vi "GEA2 Script Test SLB.vi"(0 "GEA2 Reference In":refnum<k24>, 1 "Version Query (for log header)":T2={"Source"=228, "Destination"=0, "Command"=1, "Message"=""} {"Command" format="%02x"; "Destination" format="%02x"; "Source" format="%02x"}, 2 "Enqueue Sends?":bool, 5 "Standalone":bool, 7 "Script path":path, 9 "Log File Path (empty for prompt)":path, 11 "Error In":errorcluster) -> (4 "GEA2 Reference Out":refnum<k24>, 6 "Pass/Fail?":bool, 8 "Report Text":string, 15 "Error Out":errorcluster)   [LabVIEW 2014]
doc: "This VI measures the time between the double line break closing and a burner relay closing."
uses:
  C:/Automation/DLLs/PC Tools .NET/GeaCommunication.dll
  Automation/DLLs/PC Tools .NET/GeaCommunication.dll
  type defs/Data In.ctl
  typedefs/Script Info.ctl
  type defs/Data Out.ctl
  library/GEA2_Toolkit.lvlib
panel:
  out "Script Info":T1 {"Overall Script File Progress" scale=0.0..1.0; "Elapsed time (s)" format="%#.1f"; "Current Script Progress" scale=0.0..1.0}
  in  "stop":bool
  in  "Board Index":i32
  in  "Default wait time (sec)":dbl=0.25 format="%#_13g"
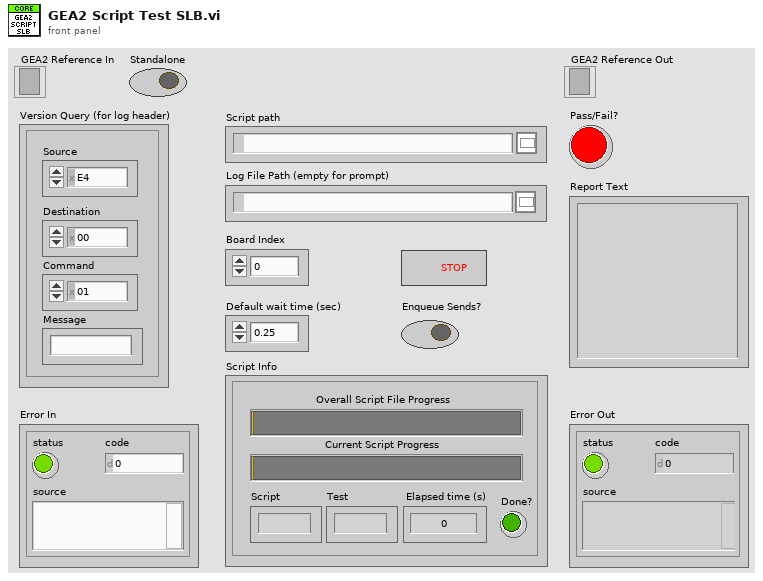
[diagram p1: front panel]
types:
  T1 = typedef "Script Info.ctl" = cluster{"Overall Script File Progress":dbl, "Current Script Progress":dbl, "Script":string, "Test":string, "Elapsed time (s)":dbl, "Done?":bool}
  T2 = typedef "GEA2_Toolkit.lvlib/Data In.ctl" = cluster{"Source":u8, "Destination":u8, "Command":u8, "Message":string}
  T3 = enum16{"open", "replace", "create", "open or create", "replace or create", "replace or create with confirmation"}
  T4 = typedef "GEA2_Toolkit.lvlib/Data Out.ctl" = cluster{"Source":u8, "Destination":u8, "Command":u8, "Length":u8, "CRC":u16, "Message":string}
  T5 = typedef "Script Output.ctl" = cluster{"Command Data":string[], "Command Type":T6[], "Test Name":string, "Wait Time (s)":dbl[], "Continue if failed?":bool[]}
  T6 = typedef "Command Type.ctl" = enum16{"WRITE", "READ", "ERDWRITE", "ERDREAD"}
  T7 = typedef "GEA2_Toolkit.lvlib/Source_Destination.ctl" = cluster{"Source":u8, "Destination":u8}
  T8 = typedef "GEA2_Toolkit.lvlib/ERD Write Data In.ctl" = cluster{"ERD Number":u16, "Data Type":enum16{"string", "boolean", "uint8_t", "uint16_t", "uint32_t"}, "Data":string}
  T9 = typedef "GEA2_Toolkit.lvlib/ERD Read Data In.ctl" = cluster{"ERD Number":u16, "Data Type":enum16{"string", "boolean", "uint8_t", "uint16_t", "uint32_t", "uint64_t"}}
  T10 = typedef "GEA2_Toolkit.lvlib/ERD Read Data Out.ctl" = cluster{"ERD Number":u16, "Data":string}
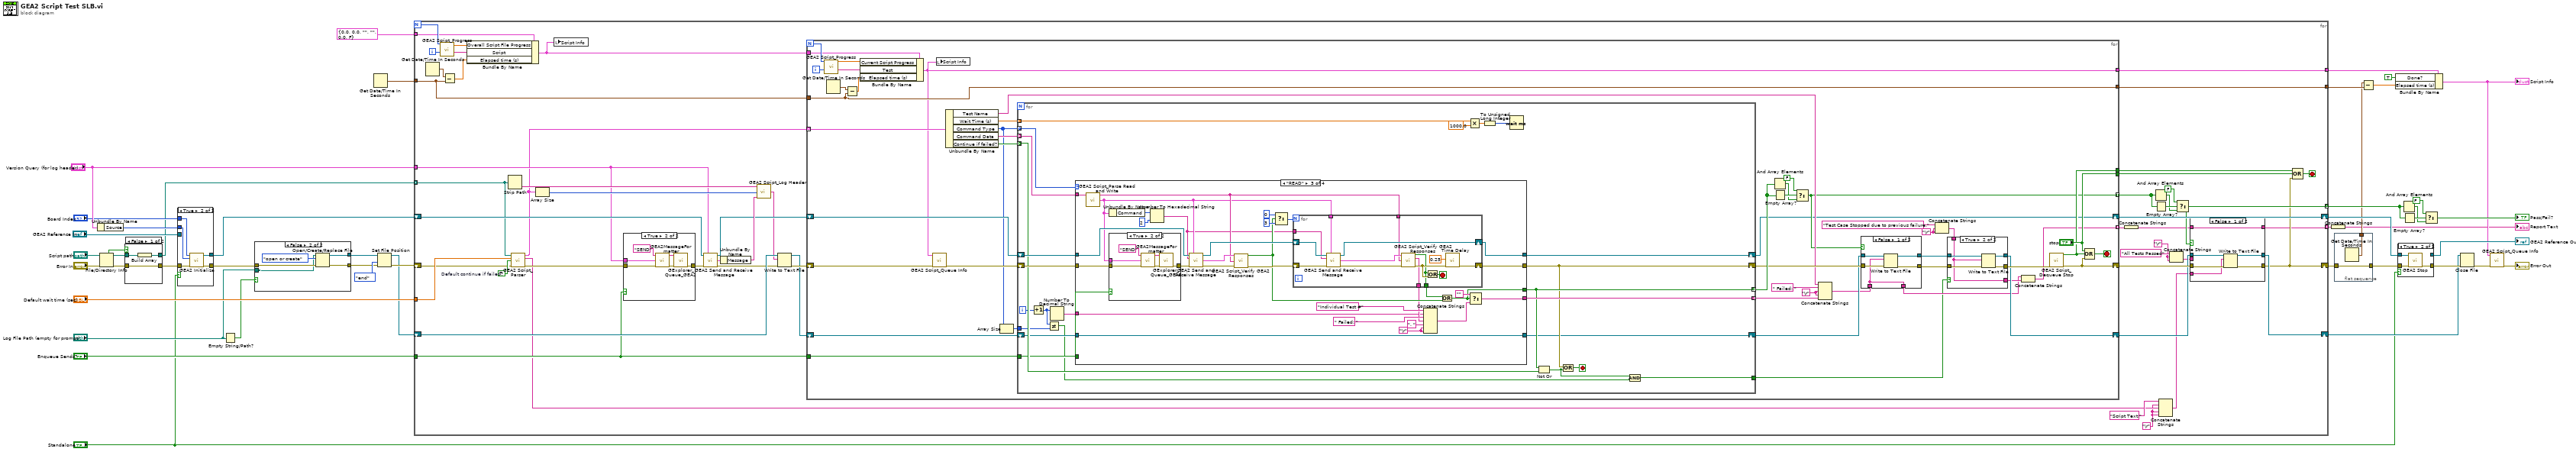
[diagram p0: block diagram]
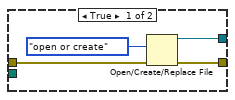
[diagram p2: hidden frame]
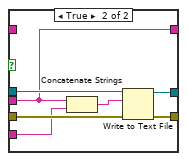
[diagram p4: hidden frame]
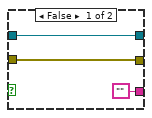
[diagram p5: hidden frame]
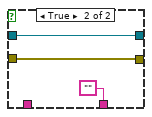
[diagram p6: hidden frame]
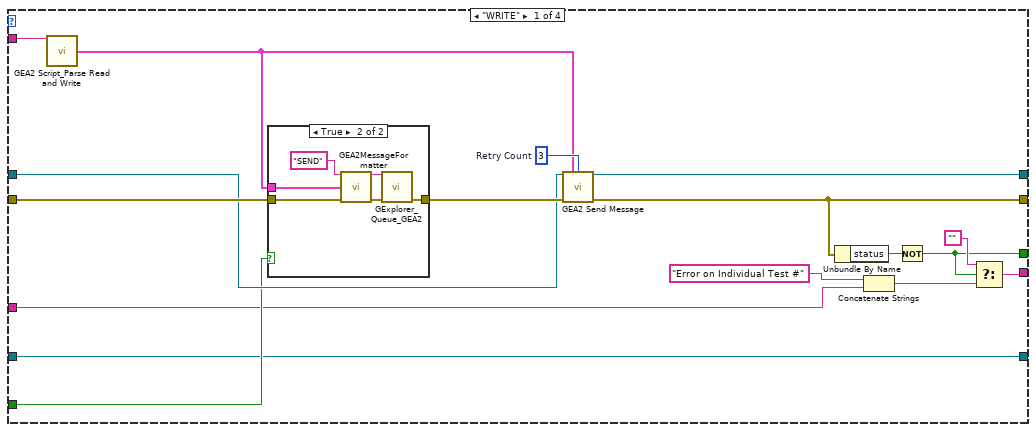
[diagram p7: hidden frame]
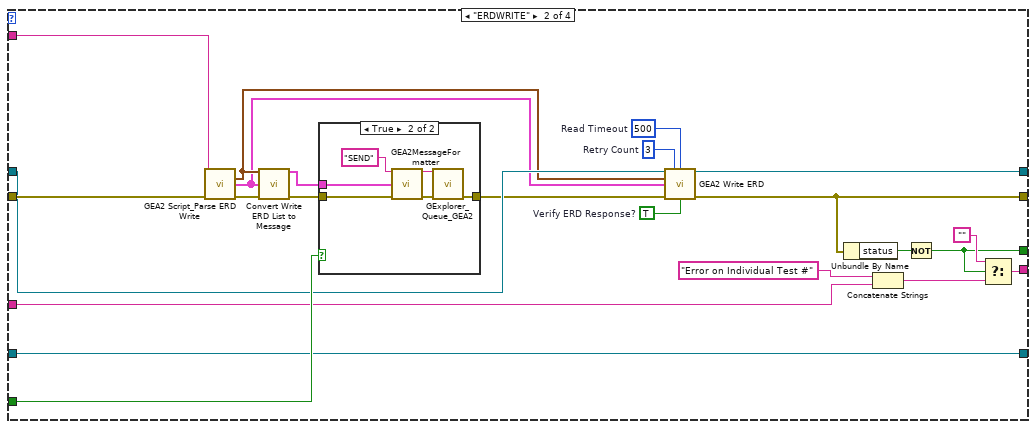
[diagram p9: hidden frame]
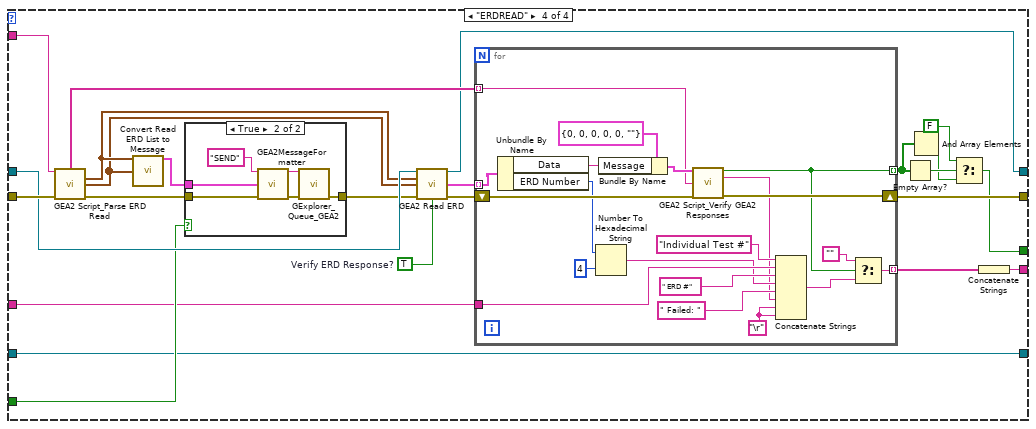
[diagram p12: hidden frame]
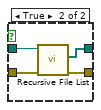
[diagram p15: hidden frame]
diagram:
  n1 = Unbundle By Name("Version Query (for log header)") -> ("Source"=w37:u8)
  n2 = File/Directory Info(path="Script path", error in="Error In") -> (path out=w41:path, directory=w40:bool, error out=w42:errorcluster)  [unwired: 4 out]
  n3 = case shown="False" w40 {
    tunnel: w42 -> [w47 w53]
    tunnel: w41 -> [w49 w52]
    tunnel: [w48 w51] -> w35
    tunnel: [w47 w50] -> w39
    frame False {
      n4 = Build Array(w49) -> (w48:path[])
    }
    frame True {
      n5 = call <vilib>:"Recursive File List.vi"("error in (no error)"=w53, "Folder Path"=w52) -> ("error out"=w50:errorcluster, "All Files in Dir"=w51:path[])  [unwired: 5 in, 3 out]
    }
  }
  n6 = case shown="True" "Standalone" {
    tunnel: [w55 w60] -> w29
    tunnel: [w54 w59] -> w32
    tunnel: "Board Index" -> [_ w57]
    tunnel: w37 -> [_ w58]
    tunnel: w39 -> [w55 w56]
    tunnel: "GEA2 Reference In" -> [w54 _]
    frame False {
    }
    frame True {
      n7 = call "GEA2 Initialize.vi"("Board Index"=w57, "Source Address"=w58, "error in"=w56) -> ("GEA2 Reference Out"=w59:refnum<k24>, "error out"=w60:errorcluster)  [unwired: 10 in, 1 out]
    }
  }
  n8 = Empty String/Path?(string/path="Log File Path (empty for prompt)") -> (empty?=w30:bool)
  n9 = case shown="False" w30 {
    tunnel: w29 -> [w63 w68]
    tunnel: [w62 w67] -> w27
    tunnel: [w61 w66] -> w26
    tunnel: "Log File Path (empty for prompt)" -> [_ w65]
    frame True {
      n10 = Open/Create/Replace File(error in=w63, operation (0:open)=T3."open or create") -> (refnum out=w62:refnum<file>, error out=w61:errorcluster)  [unwired: 4 in, 1 out]
    }
    frame False {
      n11 = Open/Create/Replace File(file path (use dialog)=w65, error in=w68, operation (0:open)=T3."open or create") -> (refnum out=w67:refnum<file>, error out=w66:errorcluster)  [unwired: 3 in, 1 out]
    }
  }
  n12 = Get Date/Time In Seconds() -> (seconds since 1Jan1904=w14:timestamp)
  n13 = Set File Position(refnum=w27, from (0:start)=enum16{"start", "end", "current"}."end", error in=w26) -> (refnum out=w24:refnum<file>, error out=w25:errorcluster)  [unwired: 1 in]
  n14 = for {
    N -> [w86]
    tunnel: "Default wait time (sec)" -> [w123]
    tunnel: "Version Query (for log header)" -> [w92]
    shift-right: [w91] -> w13
    shift-left: w25 -> [w116]
    shift-right: [w106] -> w33
    shift-left: w32 -> [w114]
    tunnel: w35 -> [w113] mode=indexing
    tunnel: "Enqueue Sends?" -> [w107]
    shift-right: [w103] -> w21
    shift-left: w24 -> [w112]
    tunnel: [w93] -> w17 mode=indexing
    tunnel: T1 {"Overall Script File Progress"=0.0, "Current Script Progress"=0.0, "Script"="", "Test"="", "Elapsed time (s)"=0.0, "Done?"=FALSE} ("Script Info") -> [w85]
    tunnel: w14 -> [w80]
    tunnel: [w79] -> w11
    tunnel: [w78] -> w9
    tunnel: [w73] -> w3 mode=indexing
    i -> [w87]
    stop <- w90 stop-if-true
    w74 = "\r"
    w70 = "\r"
    w117 = TRUE  # Default continue if failed?
    n15 = Get Date/Time In Seconds() -> (seconds since 1Jan1904=w84:timestamp)
    n16 = call "GEA2 Script_Progress.vi"("Total iterations"=w86, "Current iteration"=w87) -> ("Completion percent"=w82:dbl, "Current test"=w81:string)  [unwired: 12 in]
    n17 = Subtract(x=w84, y=w80) -> (x-y=w83:dbl)
    n18 = Bundle By Name(cluster=w85, "Overall Script File Progress"=w82, "Script"=w81, "Elapsed time (s)"=w83) -> (w77:T1)
    n19 = Strip Path(path=w113) -> (name=w122:string)  [unwired: 1 out]
    n20 = call "GEA2 Script_Parser.vi"("Script path"=w113, "Default wait time (sec)"=w123, "Default continue if failed?"=w117, "Error In"=w116) -> ("Script Output"=w71:T5[], "GEA2 Script"=w101:string, "Error Out"=w115:errorcluster)  [unwired: 9 in]
    n21 = Array Size(array=w71) -> (size(s)=w121:i32)
    n22 = local write "Script Info"(w77) -> ()
    n23 = case shown="True" w107 {
      tunnel: w92 -> [_ w386]
      tunnel: [w383 w385] -> w120
      tunnel: w115 -> [w383 w384]
      frame False {
      }
      frame True {
        n24 = call "GEA2MessageFormatter.vi"("Prefix(Send/Recv)"="SEND", "GEA2 Data In"=w386, "Error In"=w384) -> ("Output String"=w389:string, "Error Out"=w388:errorcluster)  [unwired: 11 in]
        n25 = call "GExplorer_Queue_GEA2.vi"("Output String"=w389, "error in (no error)"=w388) -> ("error out"=w385:errorcluster)  [unwired: 13 in]
      }
    }
    n26 = call "GEA2 Send and Receive Message.vi"("GEA2 Reference In"=w114, "Input Data"=w92, "Error In"=w120) -> ("GEA2 Reference Out"=w109:refnum<k24>, "Converted Data Out"=w119:T4, "Error Out"=w111:errorcluster)  [unwired: 9 in, 1 out]
    n27 = Unbundle By Name(w119) -> ("Message"=w118:string)
    n28 = call "GEA2 Script_Log Header.vi"("Filename"=w122, "# of Test Cases"=w121, "Version"=w118) -> ("Header"=w76:string)  [unwired: 12 in]
    n29 = Write to Text File(file (use dialog)=w112, text=w76, error in=w111) -> (refnum out=w108:refnum<file>, error out=w110:errorcluster)  [unwired: 1 in, 1 out]
    n30 = for {
      N -> [w170]
      tunnel: [w142] -> w75 mode=indexing
      tunnel: [w147] -> w96 mode=indexing
      shift-right: [w137] -> w105
      shift-left: w110 -> [w164]
      tunnel: w71 -> [w176] mode=indexing
      shift-right: [w146] -> w106
      shift-left: w109 -> [w162]
      shift-right: [w148] -> w104
      shift-left: w108 -> [w174]
      tunnel: w107 -> [w175]
      tunnel: ["stop"] -> w88
      tunnel: [w171] -> w89
      tunnel: w77 -> [w169]
      tunnel: w80 -> [w161]
      tunnel: [w161] -> w79
      tunnel: [w160] -> w78
      i -> [w141]
      stop <- w173 stop-if-true
      w151 = "\r"
      w155 = "\r"
      n31 = call "GEA2 Script_Progress.vi"("Total iterations"=w170, "Current iteration"=w141) -> ("Completion percent"=w167:dbl, "Current test"=w168:string)  [unwired: 12 in]
      n32 = Get Date/Time In Seconds() -> (seconds since 1Jan1904=w166:timestamp)
      n33 = Subtract(x=w166, y=w161) -> (x-y=w165:dbl)
      n34 = Bundle By Name(cluster=w169, "Current Script Progress"=w167, "Test"=w168, "Elapsed time (s)"=w165) -> (w160:T1)
      n35 = call "GEA2 Script_Queue Info.vi"("Script Info"=w160, "error in (no error)"=w164) -> ("error out"=w163:errorcluster)  [unwired: 13 in]
      n36 = local write "Script Info"(w160) -> ()
      n37 = Unbundle By Name(w176) -> ("Test Name"=w157:string, "Wait Time (s)"=w183:dbl[], "Command Type"=w140:T6[], "Command Data"=w184:string[], "Continue if failed?"=w182:bool[])
      n38 = Array Size(array=w140) -> (size(s)=w139:i32)
      n39 = for {
        shift-right: [w209] -> w159
        shift-left: w163 -> [w223]
        shift-right: [w214] -> w146
        shift-left: w162 -> [w222]
        tunnel: w140 -> [w224] mode=indexing
        tunnel: w184 -> [w221] mode=indexing
        tunnel: w183 -> [w218] mode=indexing
        tunnel: w182 -> [w220] mode=indexing
        tunnel: [w213] -> w181 mode=indexing
        tunnel: [w212] -> w177 mode=indexing
        tunnel: w175 -> [w219]
        shift-right: [w208] -> w158
        shift-left: w174 -> [w211]
        tunnel: w139 -> [w204]
        tunnel: [w201] -> w138
        i -> [w207]
        stop <- w210 stop-if-true
        n40 = Increment(x=w207) -> (x+1=w205:i32)
        n41 = Not Equal?(x=w205, y=w204) -> (x != y?=w203:bool)
        n42 = Number To Decimal String(number=w205) -> (decimal integer string=w206:string)  [unwired: 1 in]
        n43 = case shown="\"READ\"" w224 {
          tunnel: w223 -> [w238 w266 w289 w354]
          tunnel: w222 -> [w235 w263 w288 w353]
          tunnel: w221 -> [w241 w267 w310 w352]
          tunnel: [w231 w252 w301 w350] -> w209
          tunnel: [w240 w271 w302 w347] -> w214
          tunnel: [w226 w254 w293 w345] -> w213
          tunnel: [w228 w253 w291 w340] -> w212
          tunnel: w219 -> [w234 w264 w287 w336]
          tunnel: w211 -> [w233 w259 w286 w333]
          tunnel: [w233 w259 w286 w333] -> w208
          tunnel: w206 -> [w225 w249 w283 w332]
          frame "WRITE" {
            w239 = u32 3  # Retry Count
            n44 = call "GEA2 Script_Parse Read and Write.vi"("Data"=w241) -> ("GEA2 Message"=w237:T2)  [unwired: 13 in, 1 out]
            n45 = case shown="True" w234 {
              tunnel: w237 -> [_ w245]
              tunnel: [w242 w244] -> w236
              tunnel: w238 -> [w242 w243]
              frame False {
              }
              frame True {
                n46 = call "GEA2MessageFormatter.vi"("Prefix(Send/Recv)"="SEND", "GEA2 Data In"=w245, "Error In"=w243) -> ("Output String"=w248:string, "Error Out"=w247:errorcluster)  [unwired: 11 in]
                n47 = call "GExplorer_Queue_GEA2.vi"("Output String"=w248, "error in (no error)"=w247) -> ("error out"=w244:errorcluster)  [unwired: 13 in]
              }
            }
            n48 = call "GEA2 Send Message.vi"("GEA2 Reference In"=w235, "Input Data"=w237, "Retry Count"=w239, "Error In"=w236) -> ("GEA2 Reference Out"=w240:refnum<k24>, "Error Out"=w231:errorcluster)  [unwired: 10 in]
            n49 = Unbundle By Name(w231) -> ("status"=w232:bool)
            n50 = Concatenate Strings("Error on Individual Test #" ("string"), w225) -> (w227:string)
            n51 = Not(x=w232) -> (.not. x?=w228:bool)
            n52 = Select(t="", s=w228, f=w227) -> (s? t:f=w226:string)
          }
          frame "ERDWRITE" {
            w268 = TRUE  # Verify ERD Response?
            w269 = u32 500  # Read Timeout
            w270 = 3  # Retry Count
            n53 = call "GEA2 Script_Parse ERD Write.vi"("Data"=w267, "Error In"=w266) -> ("GEA Inputs"=w261:T7, "Write ERD List"=w260:T8[], "Error Out"=w251:errorcluster)  [unwired: 11 in]
            n54 = call "Convert Write ERD List to Message.vi"("GEA Inputs"=w261, "Write ERD List"=w260, "Error In"=w251) -> ("GEA Message"=w265:T2, "Error Out"=w250:errorcluster)  [unwired: 11 in]
            n55 = case shown="True" w264 {
              tunnel: w265 -> [_ w275]
              tunnel: [w272 w274] -> w262
              tunnel: w250 -> [w272 w273]
              frame False {
              }
              frame True {
                n56 = call "GEA2MessageFormatter.vi"("Prefix(Send/Recv)"="SEND", "GEA2 Data In"=w275, "Error In"=w273) -> ("Output String"=w278:string, "Error Out"=w277:errorcluster)  [unwired: 11 in]
                n57 = call "GExplorer_Queue_GEA2.vi"("Output String"=w278, "error in (no error)"=w277) -> ("error out"=w274:errorcluster)  [unwired: 13 in]
              }
            }
            n58 = call "GEA2 Write ERD.vi"("GEA2 Reference In"=w263, "Retry Count"=w270, "Read Timeout (ms)"=w269, "GEA Inputs"=w261, "Write ERD List"=w260, "Error In"=w262, "Verify ERD Response?"=w268) -> ("GEA2 Reference Out"=w271:refnum<k24>, "Error Out"=w252:errorcluster)  [unwired: 6 in, 1 out]
            n59 = Unbundle By Name(w252) -> ("status"=w258:bool)
            n60 = Concatenate Strings("Error on Individual Test #" ("string"), w249) -> (w255:string)
            n61 = Not(x=w258) -> (.not. x?=w253:bool)
            n62 = Select(t="", s=w253, f=w255) -> (s? t:f=w254:string)
          }
          frame "READ" {
            w284 = "\r"
            n63 = call "GEA2 Script_Parse Read and Write.vi"("Data"=w310) -> ("Expected Response"=w292:string, "GEA2 Message"=w282:T2)  [unwired: 13 in]
            n64 = case shown="True" w287 {
              tunnel: w282 -> [_ w314]
              tunnel: [w311 w313] -> w290
              tunnel: w289 -> [w311 w312]
              frame False {
              }
              frame True {
                n65 = call "GEA2MessageFormatter.vi"("Prefix(Send/Recv)"="SEND", "GEA2 Data In"=w314, "Error In"=w312) -> ("Output String"=w317:string, "Error Out"=w316:errorcluster)  [unwired: 11 in]
                n66 = call "GExplorer_Queue_GEA2.vi"("Output String"=w317, "error in (no error)"=w316) -> ("error out"=w313:errorcluster)  [unwired: 13 in]
              }
            }
            n67 = Unbundle By Name(w282) -> ("Command"=w281:u8)
            n68 = Number To Hexadecimal String(1:i16 2 ("width (-)"), 2:w281) -> (0:w279:string)
            n69 = call "GEA2 Send and Receive Message.vi"("GEA2 Reference In"=w288, "Input Data"=w282, "Expected Command"=w279, "Error In"=w290) -> ("GEA2 Reference Out"=w306:refnum<k24>, "Converted Data Out"=w309:T4, "Error Out"=w308:errorcluster)  [unwired: 8 in, 1 out]
            n70 = call "GEA2 Script_Verify GEA2 Responses.vi"("Actual Response"=w309, "Expected Response"=w292, "Error In"=w308) -> ("Pass/Fail?"=w299:bool, "Error Out"=w307:errorcluster)  [unwired: 10 in, 1 out]
            n71 = Select(t=0, s=w299, f=3) -> (s? t:f=w303:i32)
            n72 = for {
              N: w303 -> [_]
              shift-right: [w327] -> w301
              shift-left: w307 -> [w330]
              shift-right: [w328] -> w302
              shift-left: w306 -> [w329]
              tunnel: w292 -> [w323]
              tunnel: [w321] -> w295
              tunnel: w282 -> [w320]
              tunnel: [w319] -> w300
              tunnel: w279 -> [w318]
              stop <- w331 stop-if-true
              n73 = call "GEA2 Send and Receive Message.vi"("GEA2 Reference In"=w329, "Input Data"=w320, "Expected Command"=w318, "Error In"=w330) -> ("GEA2 Reference Out"=w328:refnum<k24>, "Converted Data Out"=w324:T4, "Error Out"=w325:errorcluster)  [unwired: 8 in, 1 out]
              n74 = call "GEA2 Script_Verify GEA2 Responses.vi"("Actual Response"=w324, "Expected Response"=w323, "Error In"=w325) -> ("Pass/Fail?"=w319:bool, "Report Text"=w321:string, "Error Out"=w322:errorcluster)  [unwired: 10 in]
              n75 = Or(x=w319, y=w322) -> (x .or. y?=w331:bool)
              n76 = call "Time Delay"("error in (no error)"=w322, "Delay Time (s)"=0.25) -> ("error out"=w327:errorcluster)  [unwired: 9 in]
            }
            n77 = Concatenate Strings("Individual Test #", w283, " Failed: " ("string"), w295, ". " ("string"), w284, w284) -> (w294:string)
            n78 = Or(x=w300, y=w299) -> (x .or. y?=w291:bool)
            n79 = Select(t="", s=w291, f=w294) -> (s? t:f=w293:string)
          }
          frame "ERDREAD" {
            w355 = TRUE  # Verify ERD Response?
            n80 = call "GEA2 Script_Parse ERD Read.vi"("Data"=w352, "Error In"=w354) -> ("Expected Responses"=w348:string[], "GEA Inputs"=w335:T7, "Read ERD List"=w334:T9[], "Error Out"=w339:errorcluster)  [unwired: 10 in]
            n81 = call "Convert Read ERD List to Message.vi"("GEA Inputs"=w335, "Read ERD List"=w334) -> ("GEA Message"=w338:T2)  [unwired: 12 in, 1 out]
            n82 = case shown="True" w336 {
              tunnel: w338 -> [_ w359]
              tunnel: [w356 w358] -> w337
              tunnel: w339 -> [w356 w357]
              frame False {
              }
              frame True {
                n83 = call "GEA2MessageFormatter.vi"("Prefix(Send/Recv)"="SEND", "GEA2 Data In"=w359, "Error In"=w357) -> ("Output String"=w362:string, "Error Out"=w361:errorcluster)  [unwired: 11 in]
                n84 = call "GExplorer_Queue_GEA2.vi"("Output String"=w362, "error in (no error)"=w361) -> ("error out"=w358:errorcluster)  [unwired: 13 in]
              }
            }
            n85 = call "GEA2 Read ERD.vi"("GEA2 Reference In"=w353, "GEA Inputs"=w335, "Read ERD List"=w334, "Error In"=w337, "Verify ERD Response?"=w355) -> ("GEA2 Reference Out"=w347:refnum<k24>, "ERD Data Out"=w349:T10[], "Error Out"=w351:errorcluster)  [unwired: 7 in, 1 out]
            n86 = for {
              shift-right: [w376] -> w350
              shift-left: w351 -> [w379]
              tunnel: w349 -> [w382] mode=indexing
              tunnel: w348 -> [w377] mode=indexing
              tunnel: [w366] -> w344 mode=indexing
              tunnel: w332 -> [w370]
              tunnel: [w365] -> w346 mode=indexing
              w363 = "\r"
              n87 = Unbundle By Name(w382) -> ("Data"=w378:string, "ERD Number"=w373:u16)
              n88 = Number To Hexadecimal String(1:i16 4 ("width (-)"), 2:w373) -> (0:w368:string)
              n89 = Bundle By Name(cluster=T4 {"Source"=0, "Destination"=0, "Command"=0, "Length"=0, "CRC"=0, "Message"=""} ("Actual Response"), "Message"=w378) -> (w380:T4)
              n90 = call "GEA2 Script_Verify GEA2 Responses.vi"("Actual Response"=w380, "Expected Response"=w377, "Error In"=w379) -> ("Pass/Fail?"=w366:bool, "Report Text"=w364:string, "Error Out"=w376:errorcluster)  [unwired: 10 in]
              n91 = Concatenate Strings("Individual Test #", w370, " ERD #", w368, " Failed: " ("string"), w364, w363, w363) -> (w375:string)
              n92 = Select(t="", s=w366, f=w375) -> (s? t:f=w365:string)
            }
            n93 = Empty Array?(array=w344) -> (empty?=w343:bool)
            n94 = And Array Elements(Boolean array=w344) -> (logical AND=w342:bool)
            n95 = Select(t=FALSE, s=w343, f=w342) -> (s? t:f=w340:bool)
            n96 = Concatenate Strings(w346) -> (w345:string)
          }
        }
        n97 = Multiply(x=w218, y=1000.0) -> (x*y=w216:dbl)
        n98 = To Unsigned Long Integer(number=w216) -> (unsigned 32bit integer=w215:u32)
        n99 = Wait (ms)(milliseconds to wait=w215) -> ()  [unwired: 1 out]
        n100 = Not Or(1:w220, 2:w212) -> (0:w202:bool)
        n101 = Or(x=w209, y=w202) -> (x .or. y?=w210:bool)
        n102 = Compound Arithmetic op=AND(w202, w203) -> (w201:bool)
      }
      n103 = And Array Elements(Boolean array=w177) -> (logical AND=w179:bool)
      n104 = Empty Array?(array=w177) -> (empty?=w180:bool)
      n105 = Select(t=FALSE, s=w180, f=w179) -> (s? t:f=w147:bool)
      n106 = Concatenate Strings(w157, " Failed: " ("string"), w155, w155, w181) -> (w145:string)
      n107 = case shown="False" w147 {
        tunnel: w159 -> [w197 w200]
        tunnel: w158 -> [w196 w199]
        tunnel: [w195 w199] -> w153
        tunnel: [w194 w200] -> w154
        tunnel: w145 -> [w193 _]
        tunnel: [w193 ""] -> w143
        frame False {
          n108 = Write to Text File(file (use dialog)=w196, text=w193, error in=w197) -> (refnum out=w195:refnum<file>, error out=w194:errorcluster)  [unwired: 1 in, 1 out]
        }
        frame True {
        }
      }
      n109 = Concatenate Strings("Test Case Stopped due to previous failure." ("string"), w151, w151) -> (w150:string)
      n110 = case shown="True" w138 {
        tunnel: w154 -> [w187 w192]
        tunnel: w153 -> [w186 w189]
        tunnel: [w186 w191] -> w148
        tunnel: [w187 w190] -> w149
        tunnel: w150 -> [_ w188]
        tunnel: ["" w188] -> w144
        frame False {
        }
        frame True {
          n111 = Write to Text File(file (use dialog)=w189, text=w188, error in=w192) -> (refnum out=w191:refnum<file>, error out=w190:errorcluster)  [unwired: 1 in, 1 out]
        }
      }
      n112 = Concatenate Strings(w143, w144) -> (w142:string)
      n113 = call "GEA2 Script_Dequeue Stop.vi"("error in (no error)"=w149) -> ("Stop Queue?"=w171:bool, "error out"=w137:errorcluster)  [unwired: 13 in]
      n114 = Compound Arithmetic op=OR("stop", w171, w137) -> (w173:bool)
    }
    n115 = Concatenate Strings(w75) -> (w72:string)
    n116 = And Array Elements(Boolean array=w96) -> (logical AND=w98:bool)
    n117 = Empty Array?(array=w96) -> (empty?=w99:bool)
    n118 = Concatenate Strings("Script Text:" ("string"), w70, w101, w70, w70) -> (w100:string)
    n119 = Concatenate Strings("All Tests Passed" ("text"), w74, w74) -> (w94:string)
    n120 = Select(t=FALSE, s=w99, f=w98) -> (s? t:f=w93:bool)
    n121 = case shown="False" w93 {
      tunnel: w105 -> [w129 w136]
      tunnel: [w126 w135] -> w91
      tunnel: w104 -> [w128 w134]
      tunnel: [w127 w133] -> w103
      tunnel: w94 -> [_ w130]
      tunnel: w100 -> [w125 w131]
      tunnel: [w124 w130] -> w73
      tunnel: w72 -> [w124 _]
      frame False {
        n122 = Write to Text File(file (use dialog)=w128, text=w125, error in=w129) -> (refnum out=w127:refnum<file>, error out=w126:errorcluster)  [unwired: 1 in, 1 out]
      }
      frame True {
        n123 = Concatenate Strings(w130, w131) -> (w132:string)
        n124 = Write to Text File(file (use dialog)=w134, text=w132, error in=w136) -> (refnum out=w133:refnum<file>, error out=w135:errorcluster)  [unwired: 1 in, 1 out]
      }
    }
    n125 = Compound Arithmetic op=OR(w89, w88, w91) -> (w90:bool)
  }
  n126 = Concatenate Strings(w3) -> (→"Report Text":string)
  n127 = flat-sequence {
    tunnel: [w391] -> w12
    tunnel: w13 -> [w391]
    tunnel: [w390] -> w10
    frame #0 {
      n128 = Get Date/Time In Seconds() -> (seconds since 1Jan1904=w390:timestamp)
    }
  }
  n129 = Subtract(x=w10, y=w11) -> (x-y=w8:dbl)
  n130 = Bundle By Name(cluster=w9, "Done?"=TRUE, "Elapsed time (s)"=w8) -> (w5:T1)
  "Script Info" <- w5
  n131 = case shown="True" "Standalone" {
    tunnel: [w393 w395] -> w22
    tunnel: w12 -> [w393 w396]
    tunnel: w33 -> [w392 w394]
    tunnel: [w392 _] -> w23
    frame False {
    }
    frame True {
      n132 = call "GEA2 Stop.vi"("GEA2 Reference In"=w394, "Error In"=w396) -> ("Error Out"=w395:errorcluster)  [unwired: 13 in]
    }
  }
  "GEA2 Reference Out" <- w23
  n133 = And Array Elements(Boolean array=w17) -> (logical AND=w19:bool)
  n134 = Empty Array?(array=w17) -> (empty?=w20:bool)
  n135 = Select(t=FALSE, s=w20, f=w19) -> (s? t:f=→"Pass/Fail?":bool)
  n136 = Close File(refnum=w21, error in=w22) -> (error out=w6:errorcluster)  [unwired: 1 out]
  n137 = call "GEA2 Script_Queue Info.vi"("Script Info"=w5, "error in (no error)"=w6) -> ("error out"=→"Error Out":errorcluster)  [unwired: 13 in]
